vi "Make Hardware Resist and Temp Calls.vi"(8 "error in (no error)":errorcluster, 11 "Engine Run Time Data in":T1) -> (0 "error out":errorcluster, 3 "Engine Run Time Data out":T1)   [LabVIEW 2023, in "NI 272x Resistive Simulation Custom Device Engine.lvlib"]
uses:
  NI 272x Resistive Simulation Custom Device Engine.lvlib
  <instrlib>/ni272xReferenceVIs/ni272xReferenceVIs.llb/ni272x Write Temperature 1Chan 1Samp.vi
  <instrlib>/ni272xReferenceVIs/ni272xReferenceVIs.llb/ni272x Write Resistance 1Chan 1Samp.vi
  Controls/Channel Mode.ctl
  NI 272x Resistive Simulation Custom Device Shared.lvlib
  <instrlib>/ni272xReferenceVIs/ni272xReferenceVIs.llb/ni272x Callendar-Van Dusen RTD Parameters.ctl
  Controls/Compiled HW Channel.ctl
  Controls/Compiled Connect Channel.ctl
  Controls/Compiled Engine Data.ctl
  <instrlib>/ni272xReferenceVIs/ni272xReferenceVIs.llb/ni272x Reference.ctl
  Controls/Engine Run Time Data.ctl
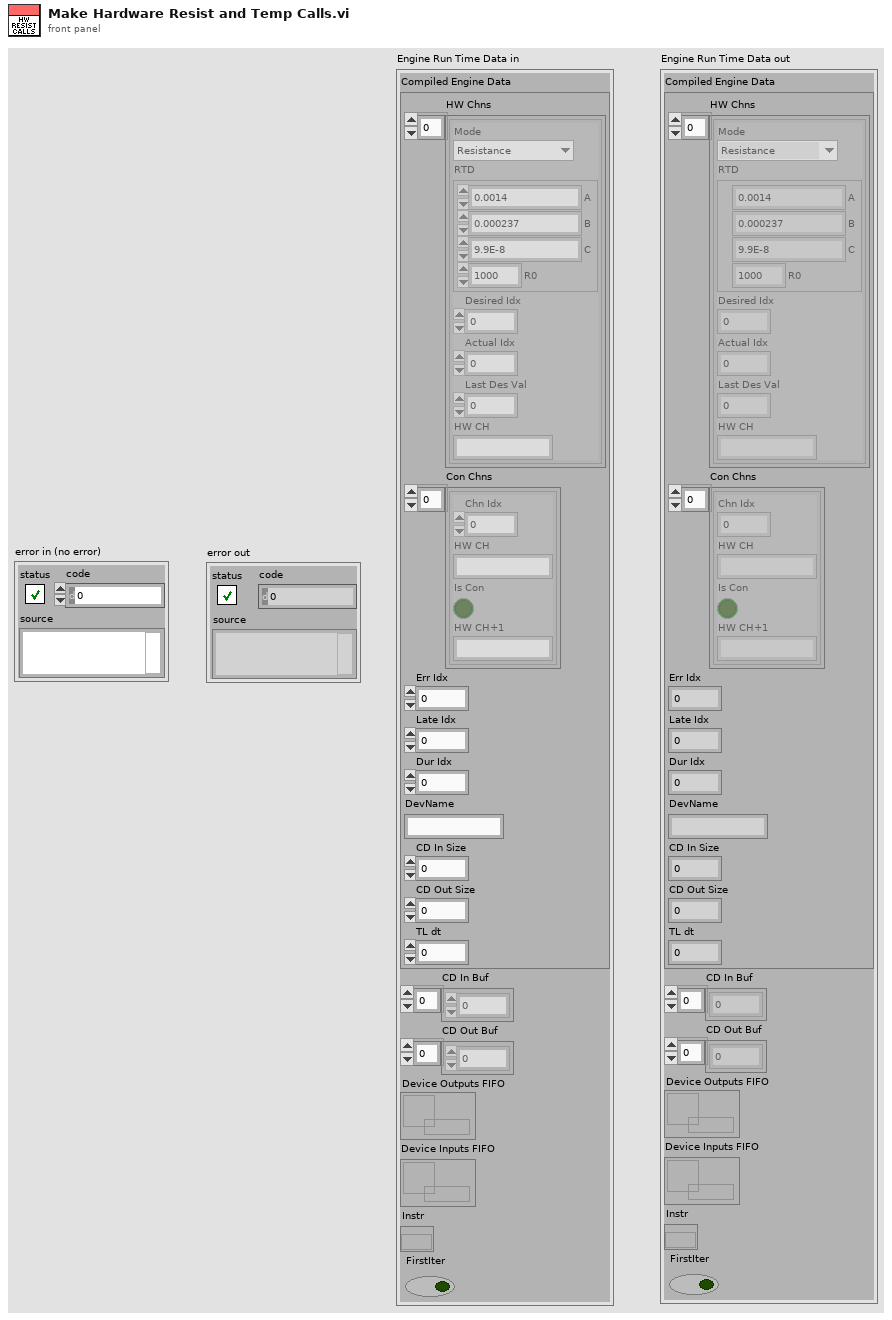
[diagram p1: front panel]
types:
  T1 = typedef "NI 272x Resistive Simulation Custom Device Engine.lvlib/Engine Run Time Data.ctl" = cluster{"Compiled Engine Data":T2, "CD In Buf":dbl[], "CD Out Buf":dbl[], "Device Outputs FIFO":refnum<k33>, "Device Inputs FIFO":refnum<k33>, "Instr":T7, "FirstIter":bool}
  T2 = typedef "NI 272x Resistive Simulation Custom Device Shared.lvlib/Compiled Engine Data.ctl" = cluster{"HW Chns":T3[], "Con Chns":T6[], "Err Idx":i32, "Late Idx":i32, "Dur Idx":i32, "DevName":string, "CD In Size":i32, "CD Out Size":i32, "TL dt":i64}
  T3 = typedef "NI 272x Resistive Simulation Custom Device Shared.lvlib/Compiled HW Channel.ctl" = cluster{"Mode":T4, "RTD":T5, "Desired Idx":i32, "Actual Idx":i32, "Last Des Val":dbl, "HW CH":string}
  T4 = typedef "NI 272x Resistive Simulation Custom Device Shared.lvlib/Channel Mode.ctl" = enum16{"Resistance", "RTD Temperature"}
  T5 = typedef "ni272x Callendar-Van Dusen RTD Parameters.ctl" = cluster{"A":dbl, "B":dbl, "C":dbl, "R0":dbl}
  T6 = typedef "NI 272x Resistive Simulation Custom Device Shared.lvlib/Compiled Connect Channel.ctl" = cluster{"Chn Idx":i32, "HW CH":string, "Is Con":bool, "HW CH+1":string}
  T7 = typedef "ni272x Reference.ctl" = refnum<k20>
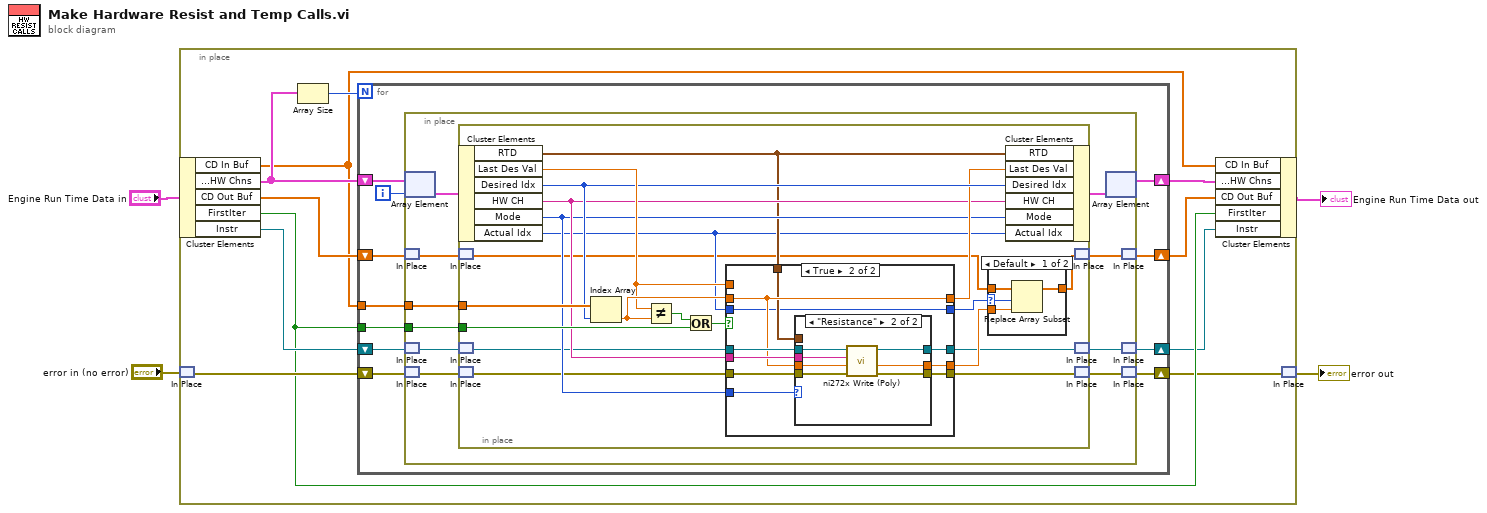
[diagram p0: block diagram]
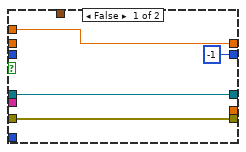
[diagram p3: hidden frame]
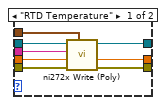
[diagram p4: hidden frame]
diagram:
  n1 = in-place {
    n2 = in-place-cluster #1("Engine Run Time Data in") -> ("CD In Buf"=w10:dbl[], "Compiled Engine Data.HW Chns"=w12:T3[], "CD Out Buf"=w11:dbl[], "FirstIter"=w7:bool, "Instr"=w15:T7)
    n3 = in-place-match #2("error in (no error)") -> (w14:errorcluster)
    n4 = Array Size(array=w12) -> (size(s)=w13:i32)
    n5 = for {
      N: w13 -> [_]
      tunnel: w10 -> [w24]
      tunnel: w7 -> [w23]
      shift-right: [w17] -> w6
      shift-left: w15 -> [w18]
      shift-right: [w19] -> w8
      shift-left: w11 -> [w20]
      shift-right: [w21] -> w5
      shift-left: w14 -> [w22]
      shift-right: [w16] -> w9
      shift-left: w12 -> [w26]
      i -> [w25]
      n6 = in-place {
        in-place-border: w24 -> [w35]
        in-place-border: w23 -> [w34]
        n7 = in-place-array #3(w26, w25) -> (w36:T3)
        n8 = in-place-match #4(w20) -> (w30:dbl[])
        n9 = in-place-match #5(w18) -> (w28:T7)
        n10 = in-place-match #6(w22) -> (w33:errorcluster)
        n11 = in-place {
          in-place-border: w35 -> [w56]
          in-place-border: w34 -> [w54]
          n12 = in-place-cluster #7(w36) -> ("RTD"=w46:T5, "Last Des Val"=w51:dbl, "Desired Idx"=w50:i32, "HW CH"=w48:string, "Mode"=w47:T4, "Actual Idx"=w42:i32)
          n13 = in-place-match #8(w30) -> (w40:dbl[])
          n14 = in-place-match #9(w28) -> (w38:T7)
          n15 = in-place-match #10(w33) -> (w44:errorcluster)
          n16 = Index Array(array=w56, index=w50) -> (element=w52:dbl)
          n17 = Not Equal?(x=w51, y=w52) -> (x != y?=w55:bool)
          n18 = Or(x=w55, y=w54) -> (x .or. y?=w53:bool)
          n19 = case shown="True" w53 {
            tunnel: w52 -> [_ w71]
            tunnel: w51 -> [w65 _]
            tunnel: [w65 w71] -> w49
            tunnel: w47 -> [_ w75]
            tunnel: w48 -> [_ w72]
            tunnel: w44 -> [w63 w74]
            tunnel: w38 -> [w62 w73]
            tunnel: w46 -> [_ w70]
            tunnel: [_ w69] -> w45
            tunnel: [w63 w68] -> w43
            tunnel: [w62 w67] -> w37
            tunnel: w42 -> [_ w66]
            tunnel: [-1 ("Actual Idx") w66] -> w41
            frame False {
            }
            frame True {
              n20 = case shown="\"Resistance\"" w75 {
                tunnel: w74 -> [w83 w90]
                tunnel: w73 -> [w82 w89]
                tunnel: w72 -> [w81 w88]
                tunnel: w71 -> [w80 w87]
                tunnel: w70 -> [w79 _]
                tunnel: [w78 w86] -> w68
                tunnel: [w77 w85] -> w67
                tunnel: [w76 w84] -> w69
                frame "RTD Temperature" {
                  n21 = call-poly <instrlib>:"ni272x Write (Poly).vi"("Callendar-Van Dusen RTD parameters"=w79, "error in (no error)"=w83, "requested temperature (degrees Celsius)"=w80, "resistor channel"=w81, "instrument handle"=w82) -> ("error out"=w78:errorcluster, "coerced temperature (degrees Celsius)"=w76:dbl, "instrument handle out"=w77:T7)  [unwired: 4 out]
                }
                frame "Resistance" {
                  n22 = call-poly <instrlib>:"ni272x Write (Poly).vi"("error in (no error)"=w90, "requested resistance (ohms)"=w87, "resistor channel"=w88, "instrument handle"=w89) -> ("error out"=w86:errorcluster, "coerced resistance (ohms)"=w84:dbl, "instrument handle out"=w85:T7)  [unwired: 1 in, 4 out]
                }
              }
            }
          }
          n23 = case shown="Default" w41 {
            selector: w41 -> [w59 _]
            tunnel: w40 -> [w60 w61]
            tunnel: w45 -> [w58 _]
            tunnel: [w57 w61] -> w39
            frame Default {
              n24 = Replace Array Subset(array=w60, new element=w58, index=w59) -> (w57:dbl[])
            }
            frame -1 {
            }
          }
          n25 = in-place-cluster #7("RTD"=w46, "Last Des Val"=w49, "Desired Idx"=w50, "HW CH"=w48, "Mode"=w47, "Actual Idx"=w42) -> (w31:T3)
          n26 = in-place-match #8(w39) -> (w29:dbl[])
          n27 = in-place-match #9(w37) -> (w27:T7)
          n28 = in-place-match #10(w43) -> (w32:errorcluster)
        }
        n29 = in-place-array #3(w31) -> (w16:T3[])  [unwired: 1 out]
        n30 = in-place-match #4(w29) -> (w19:dbl[])
        n31 = in-place-match #5(w27) -> (w17:T7)
        n32 = in-place-match #6(w32) -> (w21:errorcluster)
      }
    }
    n33 = in-place-cluster #1("CD In Buf"=w10, "Compiled Engine Data.HW Chns"=w9, "CD Out Buf"=w8, "FirstIter"=w7, "Instr"=w6) -> (→"Engine Run Time Data out":T1)
    n34 = in-place-match #2(w5) -> (→"error out":errorcluster)
  }
